vi "asAcq_dataWaitGet.vi"(0 "reference":refnum<class "OSA.lvclass">, 2 "dataType":T1, 5 "error in (no error)":errorcluster, 7 "timeout (20000 ms)":i32=20000, 9 "error if timeout":bool) -> (13 "timeOut":bool=TRUE, 14 "duplicate reference":refnum<class "OSA.lvclass">, 16 "dataType out":T1, 19 "error out":errorcluster={"status"=TRUE, "code"=1556, "source"="Thorlabs_OSA_64.lvclass:Thorlabs_OSA_64_GetAttributes.vi<ERR>\nThe reference is invalid.\n\n\n<b>Complete call chain:</b>\r\n     Thorlabs_OSA_64.lvclass:Thorlabs_OSA_64_GetAttributes.vi\r\n     Thorlabs_OSA_64.lvclass:asyncAcq_occurenceRef_timeStamp.vi\r\n     Thorlabs_OSA_64.lvclass:asyncAcq_occurenceRef_timeStamp_viServer.vi\r\n     Thorlabs_OSA_64.lvclass:asAcq_dataWait_timeStamp.vi\r\n     Thorlabs_OSA_64.lvclass:asAcq_dataWaitGet.vi"})   [LabVIEW 2010, in "OSA.lvclass"]
doc: "Waits for new data to be available and store retrieved data in a labview buffer, (see buffer_get.vi for data access)."
uses:
  OSA.lvclass
  OSA20X_misc.lvlib
  typeDef/acq_dataType.ctl
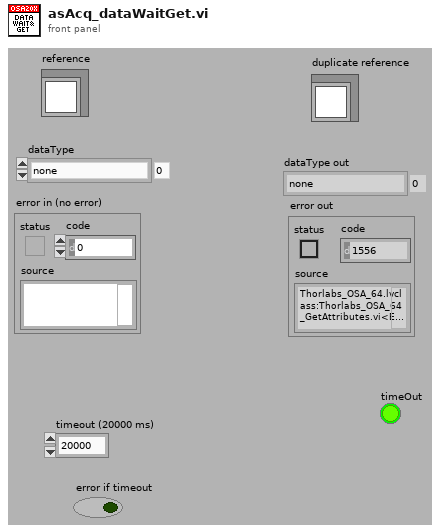
[diagram p1: front panel]
types:
  T1 = typedef "OSA.lvclass/acq_dataType.ctl" = enum16{"none", "interferogram", "spectrum"}
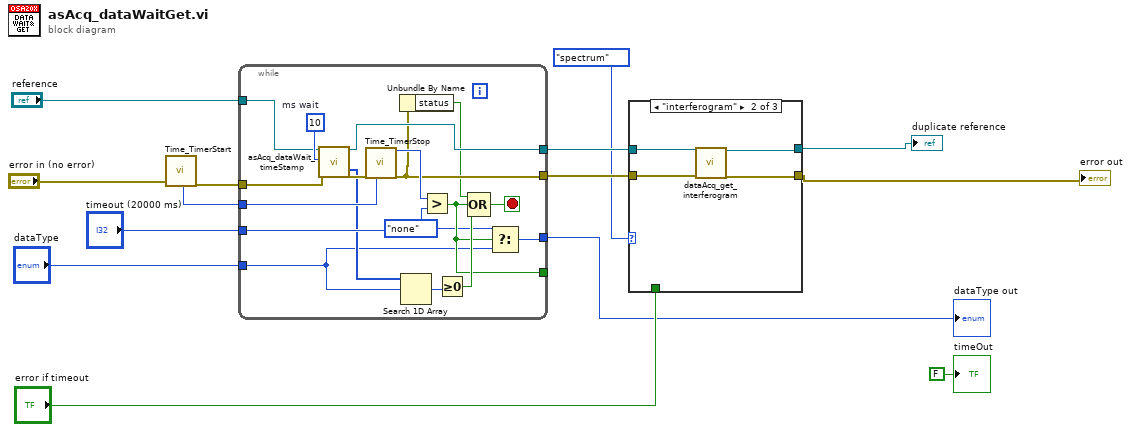
[diagram p0: block diagram]
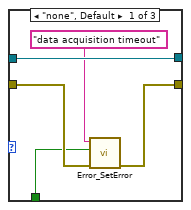
[diagram p2: hidden frame]
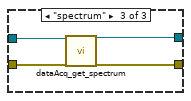
[diagram p3: hidden frame]
diagram:
  n1 = call "Time_TimerStart.vi"("error in (no error)"="error in (no error)") -> ("Start Value (ms timer)"=w11:u32, "error out"=w12:errorcluster)  [unwired: 17 in]
  n2 = while {
    tunnel: [w16] -> w14
    tunnel: [w29] -> w13
    tunnel: w12 -> [w32]
    tunnel: w11 -> [w28]
    tunnel: "timeout (20000 ms)" -> [w26]
    tunnel: "dataType" -> [w17]
    tunnel: "reference" -> [w23]
    tunnel: [w20] -> w3
    tunnel: [w19] -> _
    stop <- w22 stop-if-true
    w31 = 10  # ms wait
    n3 = call "asAcq_dataWait_timeStamp.vi"("reference"=w23, "ms wait"=w31, "error in (no error)"=w32) -> ("duplicate reference"=w29:refnum<class "OSA.lvclass">, "dataType"=w25:T1[], "error out"=w30:errorcluster)  [unwired: 14 in]
    n4 = call "Time_TimerStop.vi"("error in (no error)"=w30, "Start Value (millisecond timer)"=w28) -> ("Time (millisecond timer)"=w27:i32, "error out"=w16:errorcluster)  [unwired: 16 in]
    n5 = Unbundle By Name(w16) -> ("status"=w15:bool)
    n6 = Search 1D Array(1D array=w25, element=w17) -> (index of element=w24:i32)  [unwired: 1 in]
    n7 = Greater?(x=w27, y=w26) -> (0:w19:bool)
    n8 = Greater Or Equal To 0?(x=w24) -> (x >= 0?=w21:bool)
    n9 = Compound Arithmetic op=OR(w15, w19, w21) -> (w22:bool)
    n10 = Select(t=acq_dataType."none" ("dataType"), s=w19, f=w17) -> (s? t:f=w20:T1)
  }
  "dataType out" <- w3
  n11 = case shown="\"interferogram\"" acq_dataType."spectrum" ("dataType") {
    tunnel: w13 -> [w37 w38 w45]
    tunnel: w14 -> [w35 w41 w44]
    tunnel: [w34 w40 w43] -> w8
    tunnel: [w37 w39 w42] -> w5
    tunnel: "error if timeout" -> [w33 _ _]
    frame "none", Default {
      n12 = call "Error_SetError.vi"("error in"=w35, "status (true)"=w33, "source(\"\")"="data acquisition timeout" ("source(\"\")")) -> ("error out"=w34:errorcluster)  [unwired: 4 in]
    }
    frame "interferogram" {
      n13 = call-dynamic "dataAcq_get_interferogram.vi"("reference"=w38, "error in (no error)"=w41) -> ("duplicate reference"=w39:refnum<class "OSA.lvclass">, "error out"=w40:errorcluster)  [unwired: 16 in]
    }
    frame "spectrum" {
      n14 = call "dataAcq_get_spectrum.vi"("reference"=w45, "error in (no error)"=w44) -> ("duplicate reference"=w42:refnum<class "OSA.lvclass">, "error out"=w43:errorcluster)  [unwired: 16 in]
    }
  }
  "error out" <- w8
  "duplicate reference" <- w5
  "timeOut" <- FALSE ("timeOut")
